vi "_get_rep_cap_error.vi"(5 "Attribute":T1={"Identifier"="", "Descriptive Name"="", "Data Type"=enum."Integer 32", "Command"="", "Access"=enum."Read/Write", "Range Table"="", "Read Callback"="", "Write Callback"="", "Supported Models"="", "Instrument Options"="", "Index"=0, "OPC Wait"=FALSE, "No Status Check"=FALSE, "Cache Only"=FALSE}, 7 "Defined RepCapNames in":string[](array[string]), 8 "error in":errorcluster caption="error in (no error)", 10 "Repeated Capability":string, 11 "VISA resource name":refnum<visa-resource-name>) -> (0 "error out":errorcluster, 3 "VISA resource name out":refnum<visa-resource-name>)   [LabVIEW 2020, in "Rohde&Schwarz RTx Oscilloscopes.lvlib" / "rsidr_core.lvlib"]
uses:
  rsidr_core.lvlib
  type_Attribute.ctl
  type_Attribute_Data_Type.ctl
  type_ReadWriteAccess.ctl
  _type_Operation_Fgv_RepCap.ctl
  type_Error_Codes.ctl
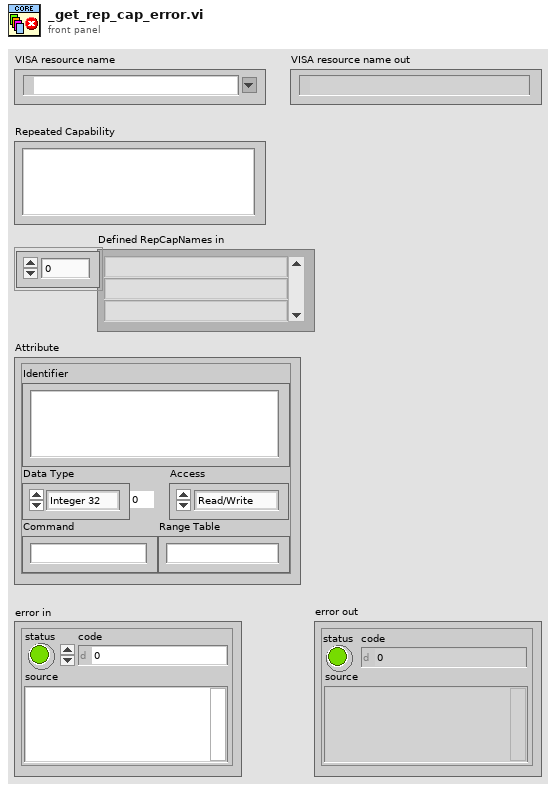
[diagram p1: front panel]
types:
  T1 = typedef "Rohde&Schwarz RTx Oscilloscopes.lvlib/rsidr_core.lvlib/type_Attribute.ctl" = cluster{"Identifier":string, "Descriptive Name":string, "Data Type":T2, "Command":string, "Access":T3, "Range Table":string, "Read Callback":string, "Write Callback":string, "Supported Models":string, "Instrument Options":string, "Index":i32, "OPC Wait":bool, "No Status Check":bool, "Cache Only":bool}
  T2 = typedef "Rohde&Schwarz RTx Oscilloscopes.lvlib/rsidr_core.lvlib/type_Attribute_Data_Type.ctl" = enum16{"Integer 32", "Double", "String", "Boolean", "None", "Integer 64", "RawString"}
  T3 = typedef "Rohde&Schwarz RTx Oscilloscopes.lvlib/rsidr_core.lvlib/type_ReadWriteAccess.ctl" = enum16{"Read Only", "Write Only", "Read/Write"}
  T4 = typedef "Rohde&Schwarz RTx Oscilloscopes.lvlib/rsidr_core.lvlib/_type_Operation_Fgv_RepCap.ctl" = enum16{"Initialize", "Get Cmd Value", "Reset Rep Cap", "Add Rep Cap", "Remove Rep Cap", "Get Rep Cap ID range", "Get Count", "Clear", "Find Name from NameID", "Get First NameID"}
  T5 = typedef "Rohde&Schwarz RTx Oscilloscopes.lvlib/rsidr_core.lvlib/type_Error_Codes.ctl" = enum16{"No_error", "VISA_err_ResourceNotFound", "VISA_err_Timeout", "VISA_warn_MoreDataAvailable", "RS_err_MissingCallback", "RS_err_InvalidAttribute", "RS_err_InvalidValue", "RS_err_UnknownResource", "RS_err_AlreadyInitialized", "RS_err_InstrumentStatus", "RS_err_BadRepCapName", "RS_err_TypesMismatch", "RS_err_ValueNotSupported", "RS_err_InvalidRngTable", "RS_err_IDqueryFail", "RS_err_UnexpResponse", "VISA_warn_ConfigNotLoaded", "RS_err_AttributeNotReadable", "RS_err_AttributeNotWritable", "RS_err_InstrumentType", "RS_err_InstrumentOption", "VISA_err_InvalidSize", "RS_err_ReliabilityIndicator", "VISA_warn_UnknownStatus", "VISA_warn_TermCharRead", "VISA_err_IO_error", "RS_err_FunctionNotSupported", "VISA_warn_QueueEmpty"}
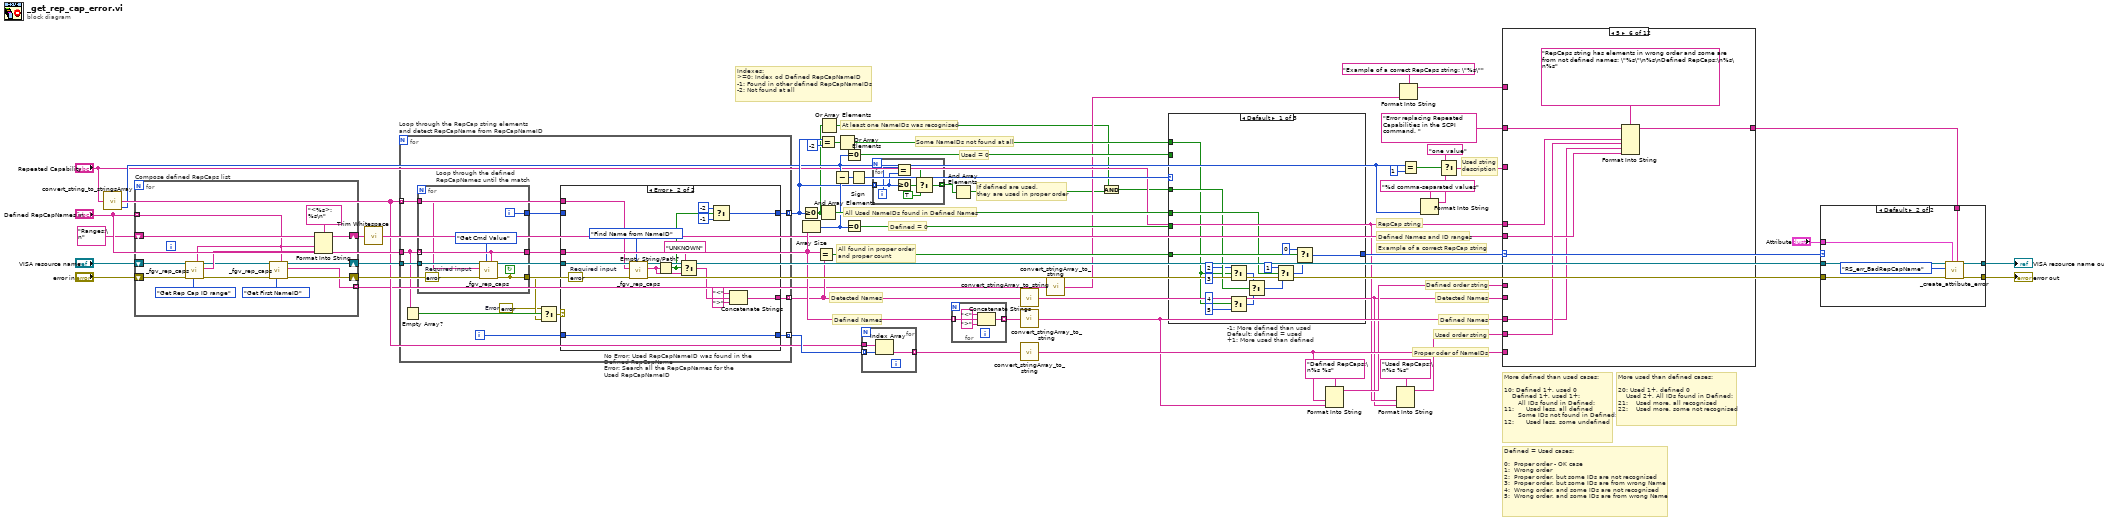
[diagram p0: block diagram]
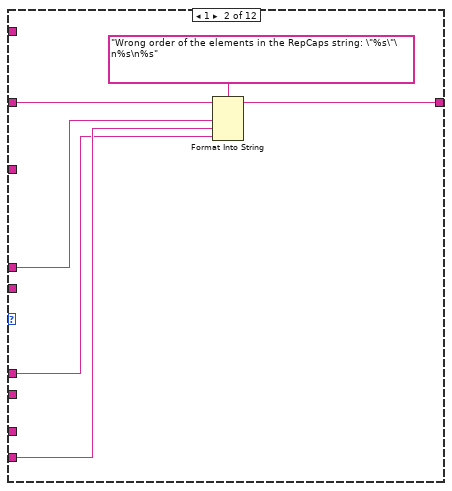
[diagram p4: hidden frame]
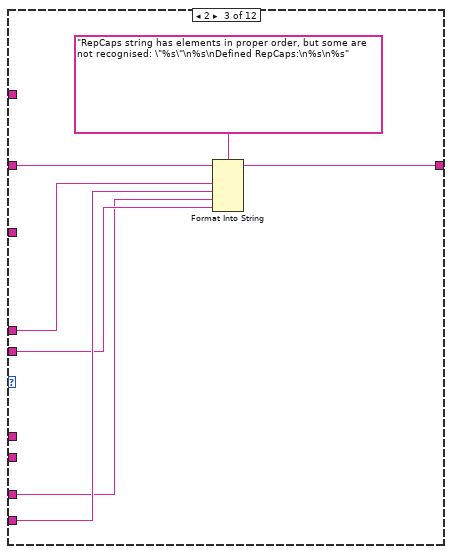
[diagram p5: hidden frame]
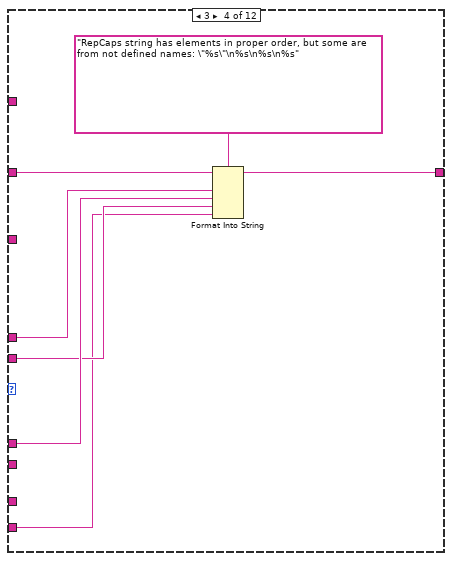
[diagram p6: hidden frame]
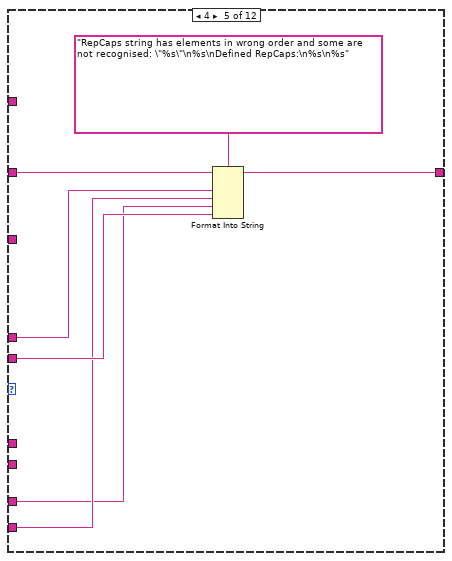
[diagram p7: hidden frame]
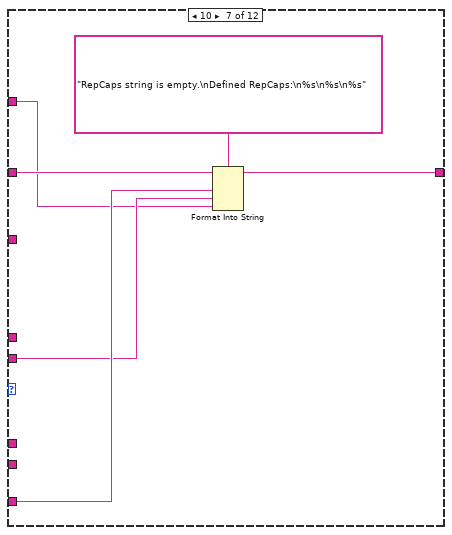
[diagram p8: hidden frame]
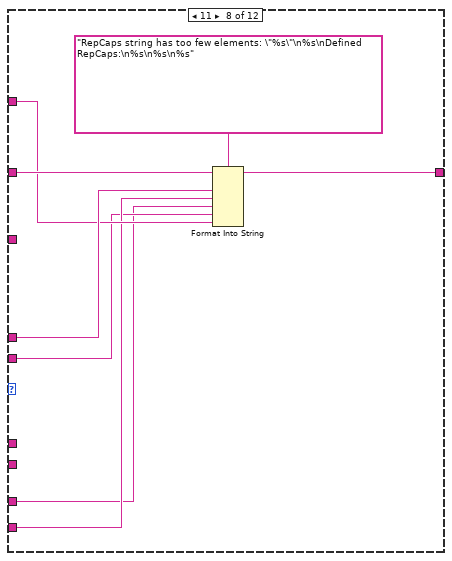
[diagram p9: hidden frame]
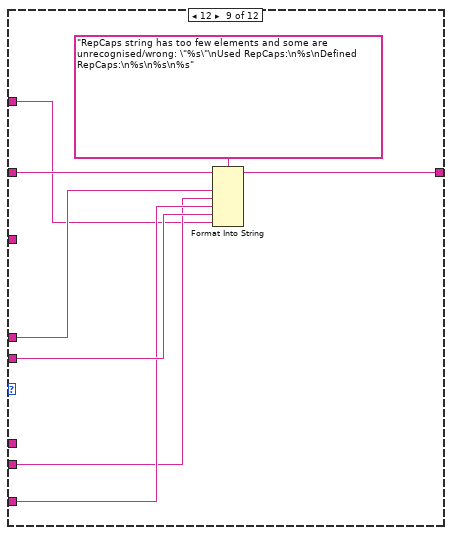
[diagram p10: hidden frame]
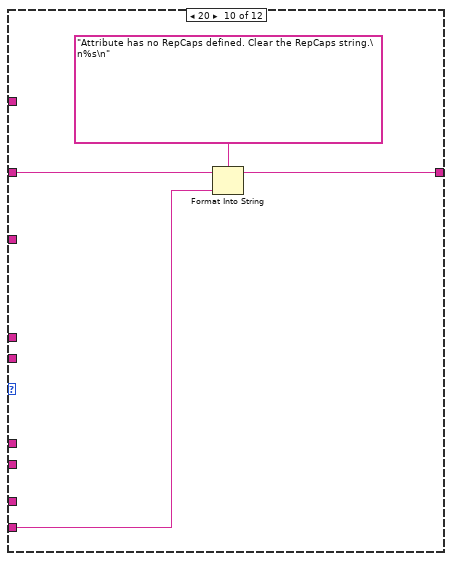
[diagram p11: hidden frame]
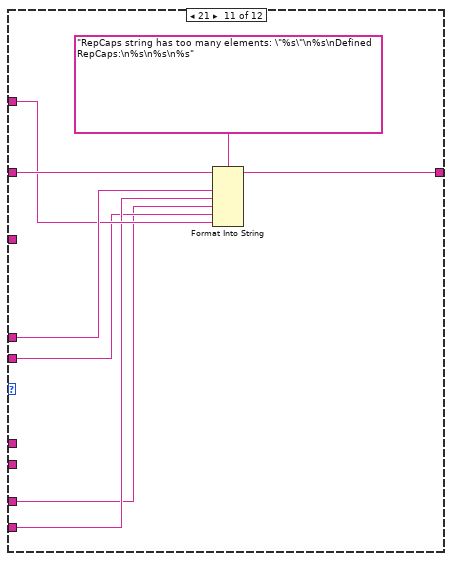
[diagram p12: hidden frame]
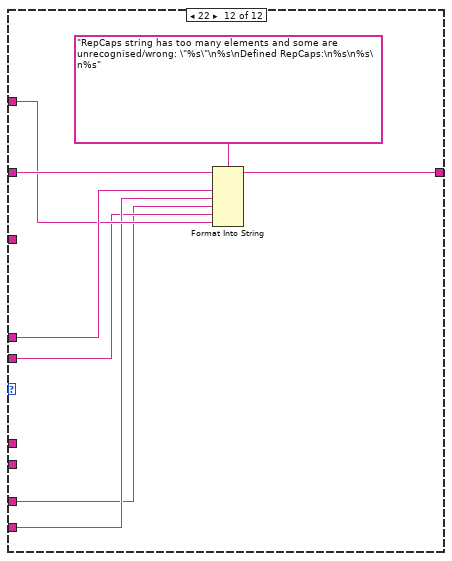
[diagram p13: hidden frame]
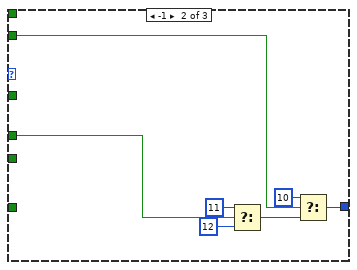
[diagram p14: hidden frame]
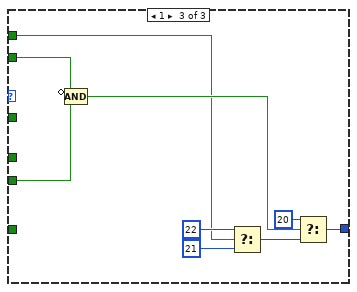
[diagram p15: hidden frame]
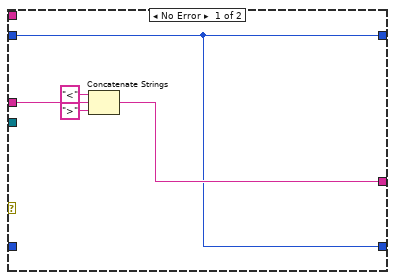
[diagram p16: hidden frame]
diagram:
  # "At least one NameIDs was recognised"
  # "Indexes:\n>=0: Index od Defined RepCapNameID\n-1: Found in other defined RepCapNameIDs\n-2: Not found at all"
  # "Used string\ndescription"
  # "Example of a correct RepCap string"
  # "Used order string"
  # "Defined order string"
  # "Proper oder of NameIDs"
  # "RepCap string"
  # "Defined Names and ID ranges"
  # "Defined Names"
  # "Detected Names"
  # "Defined Names"
  # "Defined = 0"
  # "Used = 0"
  # "If defined are used,\nthey are used in proper order"
  # "More used than defined cases:\n\n20: Used 1+, defined 0\n    Used 2+, All IDs found in Defined:\n21:    Used more, all recognised\n22:    Used more, some not recognised"
  # "Defined = Used cases:\n\n0:  Proper order - OK case\n1:  Wrong order\n2:  Proper order, but some IDs are not recognised\n3:  Proper order, but some IDs are from wrong Name\n4:  Wrong order, and some IDs are not recognised\n5:  Wrong order, and some IDs are from wrong Name"
  # "More defined than used cases:\n\n10: Defined 1+, used 0\n    Defined 1+, used 1+:\n       All IDs found in Defined:\n11:      Used less, all defined\n       Some IDs not found in Defined:\n12:      Used less, some undefined"
  # "Some NameIDs not found at all"
  # "All found in proper order\nand proper count"
  # "All Used NameIDs found in Defined Names"
  # "Detected Names"
  n1 = call "convert_string_to_stringsArray.vi"("String in"="Repeated Capability") -> ("string array size out"=w24:i32, "string array out"=w25:string[])  [unwired: 3 in]
  n2 = for "Compose defined RepCaps list" {
    shift-right: [w59] -> w41
    shift-left: "error in" -> [w68]
    shift-right: [w65] -> w27
    shift-left: "Ranges:\n" -> [w64]
    tunnel: "Defined RepCapNames in" -> [w57] mode=indexing
    shift-right: [w60] -> w40
    shift-left: "VISA resource name" -> [w67]
    tunnel: [w58] -> w9 mode=indexing
    n3 = call "_fgv_rep_caps.vi"("RepCapName in (\"\")"=w57, "Operation"=_type_Operation_Fgv_RepCap."Get Rep Cap ID range", "error in"=w68, "VISA resource name"=w67) -> ("error out"=w62:errorcluster, "CmdValue out"=w63:string, "VISA resource name out"=w61:refnum<visa-resource-name>)  [unwired: 4 in, 1 out]
    n4 = call "_fgv_rep_caps.vi"("RepCapName in (\"\")"=w57, "Operation"=_type_Operation_Fgv_RepCap."Get First NameID", "error in"=w62, "VISA resource name"=w61) -> ("error out"=w59:errorcluster, "CmdValue out"=w58:string, "VISA resource name out"=w60:refnum<visa-resource-name>)  [unwired: 4 in, 1 out]
    n5 = Format Into String(format string="<%s>: %s\n", initial string=w64, w57, w63) -> (resulting string=w65:string)  [unwired: 1 in, 1 out]
  }
  n6 = call "Trim Whitespace.vi"("string"=w27) -> ("trimmed string"=w26:string)  [unwired: 1 in]
  n7 = for "Loop through the RepCap string elements\nand detect RepCapName from RepCapNameID" {
    tunnel: w40 -> [w77]
    tunnel: w25 -> [w76] mode=indexing
    tunnel: [w81] -> w10 mode=indexing
    tunnel: [w78] -> w29 mode=indexing
    tunnel: "Defined RepCapNames in" -> [w73]
    tunnel: [w75] -> w28 mode=indexing
    i -> [w74]
    w70 = errorcluster {"status"=TRUE, "code"=0, "source"=""}  # Error
    n8 = Empty Array?(array=w73) -> (empty?=w72:bool)
    n9 = for "Loop through the defined\nRepCapNames until the match" {
      tunnel: w77 -> [w108]
      tunnel: w76 -> [w107]
      tunnel: w73 -> [w104] mode=indexing
      tunnel: [w106] -> w71
      tunnel: [w105] -> w79
      tunnel: [w104] -> w80
      i -> [w105]
      stop <- w106 continue-if-true
      w103 = errorcluster {"status"=FALSE, "code"=0, "source"=""}  # Required input
      n10 = call "_fgv_rep_caps.vi"("RepCapName in (\"\")"=w104, "Operation"=_type_Operation_Fgv_RepCap."Get Cmd Value", "error in"=w103, "RepCapNameID in (\"\")"=w107, "VISA resource name"=w108) -> ("error out"=w106:errorcluster)  [unwired: 3 in, 3 out]
    }
    n11 = Select(t=w70, s=w72, f=w71) -> (s? t:f=w69:errorcluster)
    n12 = case "No Error: Used RepCapNameID was found in the Defined RepCapName\nError: Search all the RepCapNames for the Used RepCapNameID" shown="Error" w69 {
      tunnel: [w85 w90] -> w81
      tunnel: w79 -> [w82 _]
      tunnel: w80 -> [w86 _]
      tunnel: [w82 w96] -> w78
      tunnel: w77 -> [_ w101]
      tunnel: w76 -> [_ w99]
      tunnel: [w82 w92] -> w75
      tunnel: w74 -> [_ w92]
      frame No Error {
        n13 = Concatenate Strings("<" ("string"), w86, ">" ("string")) -> (w85:string)
      }
      frame Error {
        w100 = errorcluster {"status"=FALSE, "code"=0, "source"=""}  # Required input
        n14 = call "_fgv_rep_caps.vi"("Operation"=_type_Operation_Fgv_RepCap."Find Name from NameID", "error in"=w100, "RepCapNameID in (\"\")"=w99, "VISA resource name"=w101) -> ("CmdValue out"=w97:string)  [unwired: 4 in, 3 out]
        n15 = Empty String/Path?(string/path=w97) -> (empty?=w93:bool)
        n16 = Select(t="UNKNOWN", s=w93, f=w97) -> (s? t:f=w89:string)
        n17 = Select(t=-2, s=w93, f=-1) -> (s? t:f=w96:i32)
        n18 = Concatenate Strings("<" ("string"), w89, ">" ("string")) -> (w90:string)
      }
    }
  }
  n19 = Greater Or Equal To 0?(x=w29) -> (x >= 0?=w4:bool[])
  n20 = Array Size(array="Defined RepCapNames in") -> (size(s)=w43:i32)
  n21 = Equal?(x="Defined RepCapNames in", y=w10) -> (x = y?=w48:bool)
  n22 = Equal?(x=w29, y=-2) -> (x = y?=w51:bool[])
  n23 = And Array Elements(Boolean array=w4) -> (logical AND=w44:bool)
  n24 = Or Array Elements(Boolean array=w4) -> (logical OR=w2:bool)
  n25 = Subtract(x=w24, y=w43) -> (x-y=w50:i32)
  n26 = Or Array Elements(Boolean array=w51) -> (logical OR=w45:bool)
  n27 = Equal To 0?(x=w24) -> (x = 0?=w46:bool)
  n28 = Equal To 0?(x=w43) -> (x = 0?=w42:bool)
  n29 = Sign(1:w50) -> (0:w49:i32)
  n30 = for {
    tunnel: w25 -> [w111]
    tunnel: [w110] -> w22 mode=indexing
    tunnel: w28 -> [w109] mode=indexing
    n31 = Index Array(array=w111, index=w109) -> (element=w110:string)
  }
  n32 = for {
    tunnel: w29 -> [w116] mode=indexing
    tunnel: [w114] -> w47 mode=indexing
    i -> [w115]
    n33 = Equal?(x=w115, y=w116) -> (x = y?=w117:bool)
    n34 = Greater Or Equal To 0?(x=w116) -> (x >= 0?=w112:bool)
    n35 = Select(t=w117, s=w112, f=TRUE) -> (s? t:f=w114:bool)
  }
  n36 = for {
    tunnel: "Defined RepCapNames in" -> [w119] mode=indexing
    tunnel: [w118] -> w30 mode=indexing
    n37 = Concatenate Strings("<" ("string"), w119, ">" ("string")) -> (w118:string)
  }
  n38 = And Array Elements(Boolean array=w47) -> (logical AND=w3:bool)
  n39 = call "convert_stringArray_to_string.vi"("string array in"=w10) -> ("string out"=w15:string)  [unwired: 4 in]
  n40 = call "convert_stringArray_to_string.vi"("string array in"=w30) -> ("string out"=w19:string)  [unwired: 4 in]
  n41 = call "convert_stringArray_to_string.vi"("string array in"=w22) -> ("string out"=w20:string)  [unwired: 4 in]
  n42 = call "convert_stringArray_to_string.vi"("string array in"=w9) -> ("string out"=w6:string)  [unwired: 4 in]
  n43 = And(x=w2, y=w3) -> (x .and. y?=w1:bool)
  n44 = case "-1: More defined than used\nDefault: defined = used\n+1: More used than defined" shown="Default" w49 {
    tunnel: w48 -> [w136 _ _]
    tunnel: w44 -> [w133 w139 _]
    tunnel: w45 -> [w128 _ w145]
    tunnel: w1 -> [w130 _ _]
    tunnel: [w129 w143 w152] -> w39
    tunnel: w46 -> [_ w142 w149]
    tunnel: w42 -> [_ _ w148]
    frame Default {
      n45 = Select(t=2, s=w128, f=3) -> (s? t:f=w126:i32)
      n46 = Select(t=4, s=w128, f=5) -> (s? t:f=w127:i32)
      n47 = Select(t=w126, s=w130, f=w127) -> (s? t:f=w131:i32)
      n48 = Select(t=1, s=w133, f=w131) -> (s? t:f=w134:i32)
      n49 = Select(t=0, s=w136, f=w134) -> (s? t:f=w129:i32)
    }
    frame -1 {
      n50 = Select(t=11, s=w139, f=12) -> (s? t:f=w140:i32)
      n51 = Select(t=10, s=w142, f=w140) -> (s? t:f=w143:i32)
    }
    frame 1 {
      n52 = Compound Arithmetic op=AND(invert w149, w148) -> (w147:bool)
      n53 = Select(t=22, s=w145, f=21) -> (s? t:f=w150:i32)
      n54 = Select(t=20, s=w147, f=w150) -> (s? t:f=w152:i32)
    }
  }
  n55 = Format Into String(format string="Defined RepCaps:\n%s %s", w20, w19) -> (resulting string=w18:string)  [unwired: 2 in, 1 out]
  n56 = Format Into String(format string="Used RepCaps:\n%s %s", "Repeated Capability", w15) -> (resulting string=w14:string)  [unwired: 2 in, 1 out]
  n57 = Format Into String(format string="Example of a correct RepCaps string: \"%s\"", w6) -> (resulting string=w7:string)  [unwired: 2 in, 1 out]
  n58 = Equal?(x=w24, y=1) -> (x = y?=w34:bool)
  n59 = Format Into String(format string="%d comma-separated values", w24) -> (resulting string=w37:string)  [unwired: 2 in, 1 out]
  n60 = Select(t="one value", s=w34, f=w37) -> (s? t:f=w32:string)
  n61 = case shown="5" w39 {
    tunnel: "Error replacing Repeated Capabilities in the SCPI command. " -> [_ w158 w165 w172 w179 w186 w192 w200 w208 w212 w220 w228]
    tunnel: w32 -> [_ _ _ _ _ _ _ _ _ _ _ _]
    tunnel: w19 -> [_ _ w159 _ w173 w180 w189 w193 w203 _ w213 w221]
    tunnel: w15 -> [_ _ _ _ _ _ _ _ w202 _ _ _]
    tunnel: w26 -> [_ _ w160 w167 w177 w181 w188 w194 w204 _ w214 w222]
    tunnel: "Repeated Capability" -> [_ w155 w162 w168 w175 w183 _ w197 w205 _ w217 w225]
    tunnel: w20 -> [_ _ _ _ _ _ _ _ _ _ _ _]
    tunnel: w18 -> [_ w153 _ w169 _ _ _ _ _ _ _ _]
    tunnel: w14 -> [_ w154 w161 w166 w174 w182 _ w195 _ w209 w215 w223]
    tunnel: [_ w156 w164 w171 w178 w185 w191 w199 w207 w211 w219 w227] -> w11
    tunnel: w7 -> [_ _ _ _ _ _ w187 w196 w201 _ w216 w224]
    frame 0, Default {
    }
    frame 1 {
      n62 = Format Into String(format string="Wrong order of the elements in the RepCaps string: \"%s\"\n%s\n%s", initial string=w158, w155, w154, w153) -> (resulting string=w156:string)  [unwired: 1 in, 1 out]
    }
    frame 2 {
      n63 = Format Into String(format string="RepCaps string has elements in proper order, but some are not recognised: \"%s\"\n%s\nDefined RepCaps:\n%s\n%s", initial string=w165, w162, w161, w159, w160) -> (resulting string=w164:string)  [unwired: 1 in, 1 out]
    }
    frame 3 {
      n64 = Format Into String(format string="RepCaps string has elements in proper order, but some are from not defined names: \"%s\"\n%s\n%s\n%s", initial string=w172, w168, w169, w167, w166) -> (resulting string=w171:string)  [unwired: 1 in, 1 out]
    }
    frame 4 {
      n65 = Format Into String(format string="RepCaps string has elements in wrong order and some are not recognised: \"%s\"\n%s\nDefined RepCaps:\n%s\n%s", initial string=w179, w175, w174, w173, w177) -> (resulting string=w178:string)  [unwired: 1 in, 1 out]
    }
    frame 5 {
      n66 = Format Into String(format string="RepCaps string has elements in wrong order and some are from not defined names: \"%s\"\n%s\nDefined RepCaps:\n%s\n%s", initial string=w186, w183, w182, w180, w181) -> (resulting string=w185:string)  [unwired: 1 in, 1 out]
    }
    frame 10 {
      n67 = Format Into String(format string="RepCaps string is empty.\nDefined RepCaps:\n%s\n%s\n%s", initial string=w192, w189, w188, w187) -> (resulting string=w191:string)  [unwired: 1 in, 1 out]
    }
    frame 11 {
      n68 = Format Into String(format string="RepCaps string has too few elements: \"%s\"\n%s\nDefined RepCaps:\n%s\n%s\n%s", initial string=w200, w197, w195, w193, w194, w196) -> (resulting string=w199:string)  [unwired: 1 in, 1 out]
    }
    frame 12 {
      n69 = Format Into String(format string="RepCaps string has too few elements and some are unrecognised/wrong: \"%s\"\nUsed RepCaps:\n%s\nDefined RepCaps:\n%s\n%s\n%s", initial string=w208, w205, w202, w203, w204, w201) -> (resulting string=w207:string)  [unwired: 1 in, 1 out]
    }
    frame 20 {
      n70 = Format Into String(format string="Attribute has no RepCaps defined. Clear the RepCaps string.\n%s\n", initial string=w212, w209) -> (resulting string=w211:string)  [unwired: 1 in, 1 out]
    }
    frame 21 {
      n71 = Format Into String(format string="RepCaps string has too many elements: \"%s\"\n%s\nDefined RepCaps:\n%s\n%s\n%s", initial string=w220, w217, w215, w213, w214, w216) -> (resulting string=w219:string)  [unwired: 1 in, 1 out]
    }
    frame 22 {
      n72 = Format Into String(format string="RepCaps string has too many elements and some are unrecognised/wrong: \"%s\"\n%s\nDefined RepCaps:\n%s\n%s\n%s", initial string=w228, w225, w223, w221, w222, w224) -> (resulting string=w227:string)  [unwired: 1 in, 1 out]
    }
  }
  n73 = case shown="Default" w39 {
    tunnel: w41 -> [w230 w237]
    tunnel: w40 -> [w229 w235]
    tunnel: "Attribute" -> [_ w234]
    tunnel: [w229 w233] -> w13
    tunnel: [w230 w232] -> w12
    tunnel: w11 -> [_ w231]
    frame 0 {
    }
    frame Default {
      n74 = call "_create_attribute_error.vi"("Error Elaboration (\"\")"=w231, "Attribute"=w234, "error in"=w237, "Error Enum in"=type_Error_Codes."RS_err_BadRepCapName", "VISA resource name"=w235) -> ("error out"=w232:errorcluster, "VISA resource name out"=w233:refnum<visa-resource-name>)  [unwired: 5 in]
    }
  }
  "error out" <- w12
  "VISA resource name out" <- w13
